vi "Initialize.vi"(8 "error in":errorcluster, 10 "Device Name":string) -> (0 "error out":errorcluster, 3 "PIOD out":refnum<class "PIOD.lvclass">)   [LabVIEW 2018]
uses:
  builds/Configuration.lvlibp/Configuration.lvclass
  PIOD.lvclass
  C:/Users/Ron.Dexter.LUMINARTECH/Desktop/builds/PLC.lvlibp/PLC.lvclass
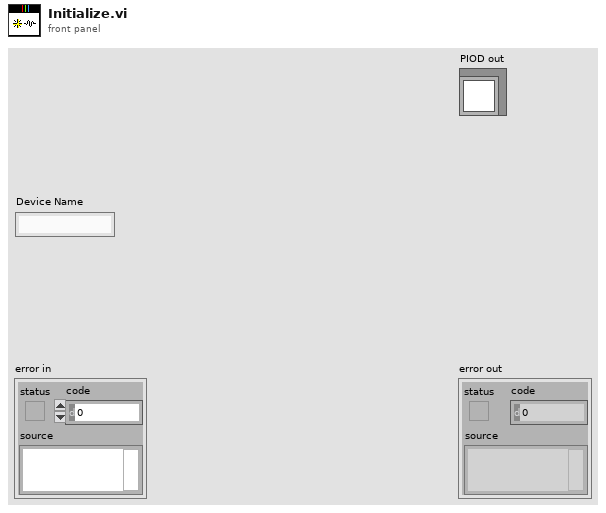
[diagram p1: front panel]
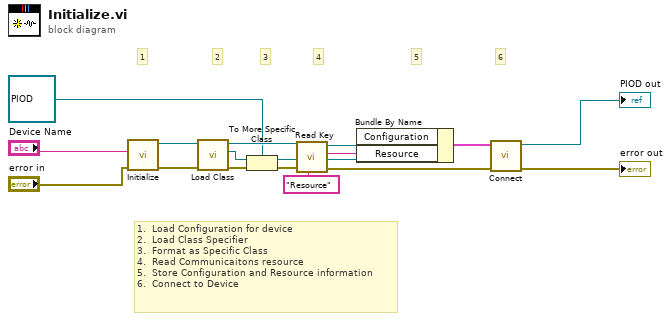
[diagram p0: block diagram]
diagram:
  # "6"
  # "1.  Load Configuration for device\n2.  Load Class Specifier\n3.  Format as Specific Class\n4.  Read Communicaitons resource\n5.  Store Configuration and Resource information\n6.  Connect to Device"
  # "5"
  # "4"
  # "3"
  # "2"
  # "1"
  n1 = call "Initialize.vi"("error in"="error in", "Device"="Device Name") -> ("error out"=w9:errorcluster, "Configuration out"=w10:refnum<class "Configuration.lvclass">)  [unwired: 8 in]
  n2 = call "Load Class.vi"("error in"=w9, "Configuration in"=w10) -> ("error out"=w15:errorcluster, "Class out"=w14:refnum<class>, "Configuration out"=w12:refnum<class "Configuration.lvclass">)  [unwired: 7 in]
  n3 = To More Specific Class(target class=refnum<class "PIOD.lvclass"> refnum ("PIOD out"), reference=w14, error in=w15) -> (specific class reference=w7:refnum<class "PIOD.lvclass">, error out=w13:errorcluster)
  n4 = call "Read Key.vi"("Key:"="Resource", "error in"=w13, "Configuration in"=w12) -> ("error out"=w1:errorcluster, "Value"=w5:string, "Configuration out"=w6:refnum<class "Configuration.lvclass">)  [unwired: 6 in]
  n5 = Bundle By Name(cluster=w7, "Configuration"=w6, "Resource"=w5) -> (w4:cluster{})
  n6 = call-dynamic "Connect.vi"("error in"=w1, "PIOD in"=w4) -> ("error out"=→"error out":errorcluster, "PIOD out"=→"PIOD out":refnum<class "PIOD.lvclass">)  [unwired: 8 in]
